vi "Read Description.vi"(11 "Assertion Result In":refnum<class "Assertion Result.lvclass">) -> (2 "Description":string, 3 "Assertion Result Out":refnum<class "Assertion Result.lvclass">)   [LabVIEW 2020, in "Assertion Result.lvclass"]
uses:
  Assertion Result.lvclass
  Assertion Result.lvclass/Assertion Result.ctl
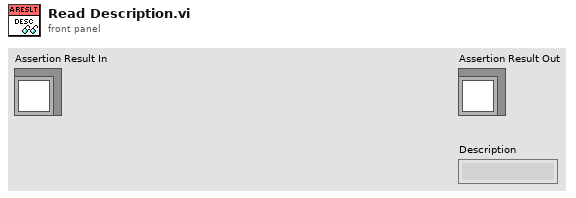
[diagram p1: front panel]
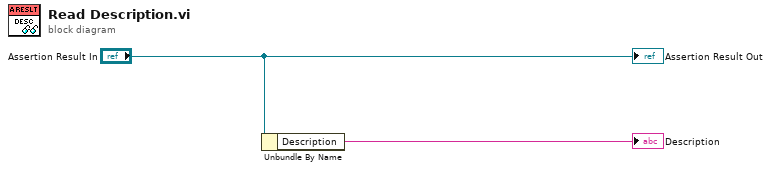
[diagram p0: block diagram]
diagram:
  n1 = Unbundle By Name("Assertion Result In") -> ("Description"=→"Description":string)
  "Assertion Result Out" <- "Assertion Result In"
